vi "vi.vi"() -> ()   [LabVIEW 2014]
uses:
  <vilib>/addons/TestStand/_TSLegacy.llb/LabVIEW Test - Invocation Info.ctl
panel:
  in  "Boolean":bool
  in  "Invocation info":T1
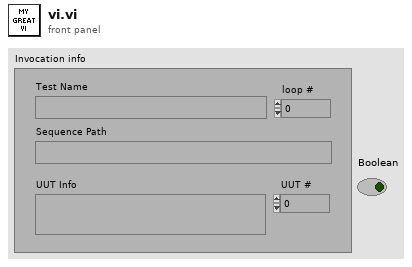
[diagram p1: front panel]
types:
  T1 = typedef "LabVIEW Test - Invocation Info.ctl" = cluster{"UUT #":i32, "loop #":i32, "UUT Info":string, "Test Name":string, "Sequence Path":path}
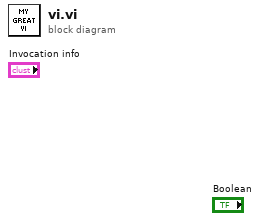
[diagram p0: block diagram]
diagram:
